vi "Function.Lookup Module Name form Function Command Prefix.vi"(9 "Function Name with Prefix":string, 10 "Other Modules":string[](array[string]), 11 "Child Modules":cluster{"Name":string, "vi ref":refnum<vi>}[](array[cluster])) -> (1 "Found":bool, 2 "Function Name":string, 3 "Module Name":string)   [LabVIEW 2019]
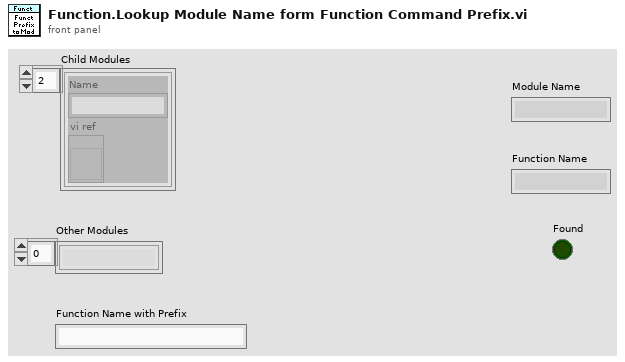
[diagram p1: front panel]
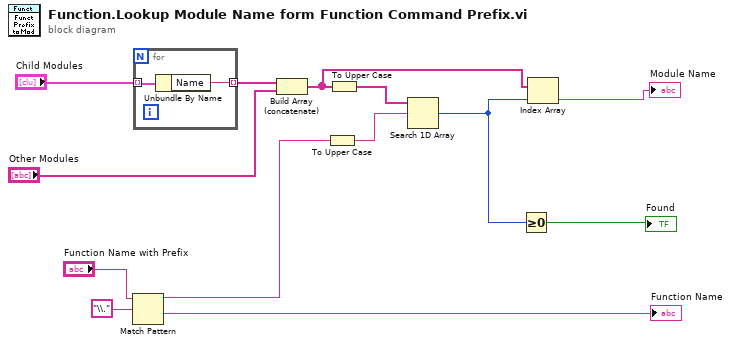
[diagram p0: block diagram]
diagram:
  n1 = Match Pattern(string="Function Name with Prefix", regular expression="\\.") -> (before substring=w7:string, after substring=→"Function Name":string)  [unwired: 1 in, 2 out]
  n2 = for {
    tunnel: "Child Modules" -> [w15] mode=indexing
    tunnel: [w14] -> w12 mode=indexing
    n3 = Unbundle By Name(w15) -> ("Name"=w14:string)
  }
  n4 = Build Array (concatenate)(w12, "Other Modules") -> (w1:string[])
  n5 = To Upper Case(1:w7) -> (0:w6:string)
  n6 = To Upper Case(1:w1) -> (0:w3:string[])
  n7 = Search 1D Array(1D array=w3, element=w6) -> (index of element=w4:i32)  [unwired: 1 in]
  n8 = Greater Or Equal To 0?(x=w4) -> (x >= 0?=→"Found":bool)
  n9 = Index Array(array=w1, index=w4) -> (element=→"Module Name":string)
